vi "GetTime.vi"(1 "error in":errorcluster) -> (0 "Time":u32)   [LabVIEW 2015]
doc: "Gets the value from the millisecond timer. Meant to be synced with an error cluster for benchmarking."
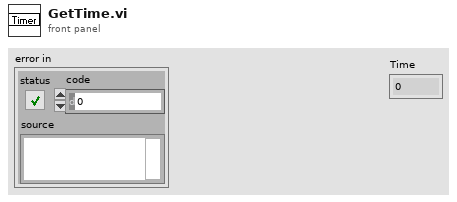
[diagram p1: front panel]
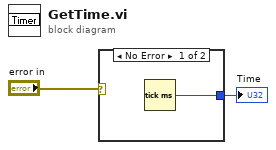
[diagram p0: block diagram]
diagram:
  n1 = case shown="No Error" "error in" {
    tunnel: [w3 _] -> w1
    frame No Error {
      n2 = Tick Count (ms)() -> (millisecond timer value=w3:u32)
    }
    frame Error {
    }
  }
  "Time" <- w1
